vi "dfd_Convert Representation to Datatype.vi"(1 "input type":T1(ring)) -> (0 "Datatype":i16)   [LabVIEW 2017, in "NI_DigFilterLicensed.lvlib"]
uses:
  <vilib>/addons/Digital Filter Design/NI_DigFilterLicensed.lvlib
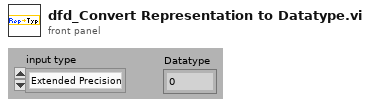
[diagram p1: front panel]
types:
  T1 = enum32{"Extended Precision", "Double Precision", "Single Precision", "Long", "Word", "Byte", "Unsigned Long", "Unsigned Word", "Unsigned Byte", "Complex Extended", "Complex Double", "Complex Single", "Quad", "Unsigned Quad"}
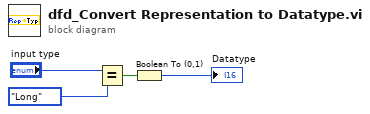
[diagram p0: block diagram]
diagram:
  n1 = Equal?(x="input type", y=T1."Long") -> (x = y?=w3:bool)
  n2 = Boolean To (0,1)(Boolean=w3) -> (0, 1=→"Datatype":i16)
